vi "BCC.vi"(3 "Message":string="\u00050ArSB08%DW1000032\u0004") -> (0 "BCC":string, 1 "Message with BCC":string="A")   [LabVIEW 2014]
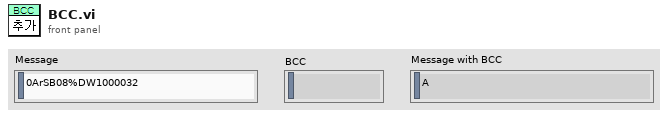
[diagram p1: front panel]
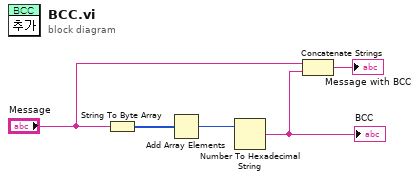
[diagram p0: block diagram]
diagram:
  n1 = String To Byte Array(string="Message") -> (unsigned byte array=w5:u8[])
  n2 = Add Array Elements(numeric array=w5) -> (sum=w4:u8)
  n3 = Number To Hexadecimal String(2:w4) -> (0:w2:string)  [unwired: 1 in]
  "BCC" <- w2
  n4 = Concatenate Strings("Message", w2) -> (→"Message with BCC":string)
